vi "Last Write Block.vi"(6 "tdms file Ref":refnum<k34>, 7 "Group Name TMDS":string, 8 "error in":errorcluster, 9 "Data":waveform(dbl)[](array[waveform]), 10 "End Block?":bool, 11 "Acq and Logging Props":T1) -> (0 "error out":errorcluster, 2 "Message":string, 3 "tdms file out":refnum<k34>)   [LabVIEW 2013]
uses:
  <vilib>/Analysis/5stat.llb/RMS (DBL).vi
  <vilib>/Analysis/NI_AALPro.lvlib
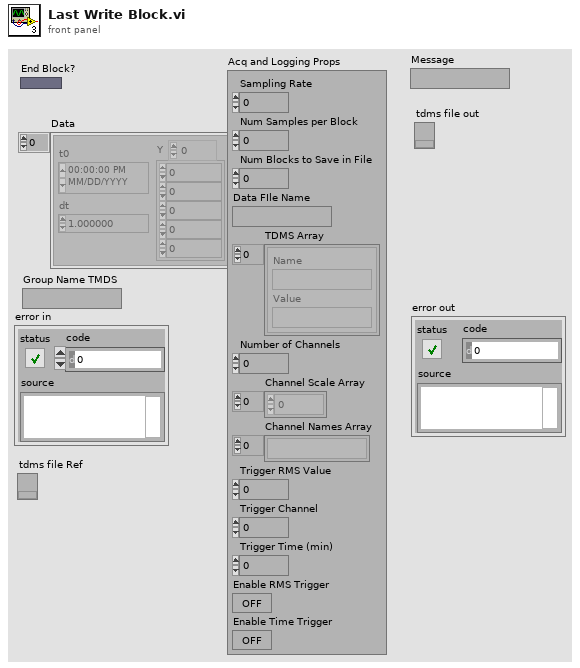
[diagram p1: front panel]
types:
  T1 = cluster{"Sampling Rate":dbl, "Num Samples per Block":i32, "Num Blocks to Save in File":i32, "Data FIle Name":string, "TDMS Array":cluster{"Name":string, "Value":string}[], "Number of Channels":i32, "Channel Scale Array":dbl[], "Channel Names Array":string[], "Trigger RMS Value":dbl, "Trigger Channel":i32, "Trigger Time (min)":i32, "Enable RMS Trigger":bool, "Enable Time Trigger":bool}
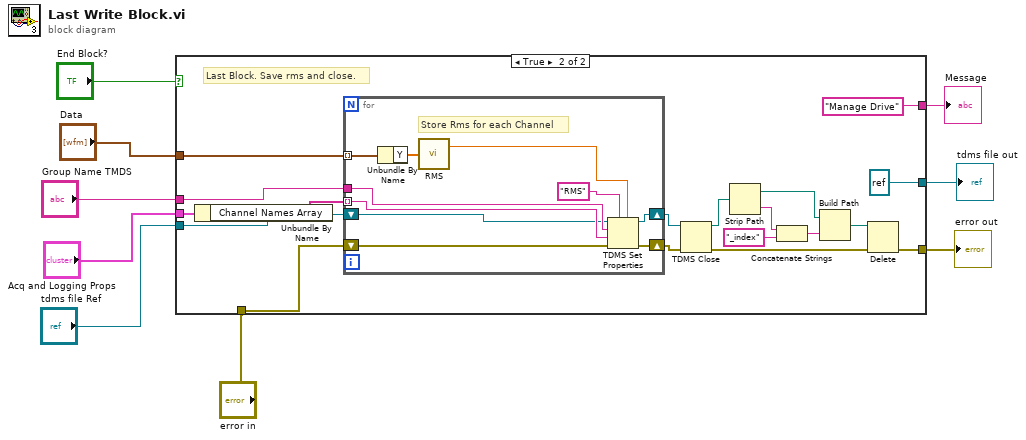
[diagram p0: block diagram]
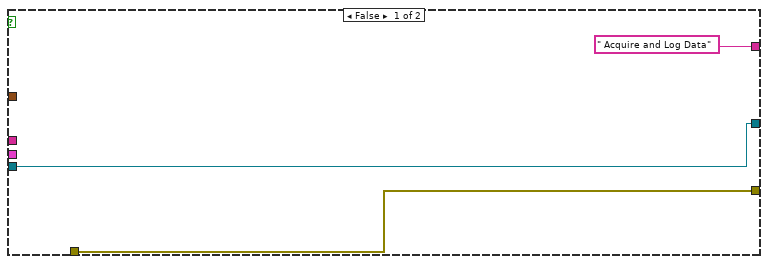
[diagram p2: hidden frame]
diagram:
  n1 = case shown="True" "End Block?" {
    tunnel: "Acq and Logging Props" -> [_ w30]
    tunnel: "Group Name TMDS" -> [_ w28]
    tunnel: "tdms file Ref" -> [w12 w27]
    tunnel: "Data" -> [_ w26]
    tunnel: [w10 w14] -> w3
    tunnel: "error in" -> [w10 w17]
    tunnel: [w12 refnum<k34> refnum ("tdms file out")] -> w2
    tunnel: [" Acquire and Log Data" ("Message") "Manage Drive" ("Message")] -> w1
    frame False {
    }
    frame True {
      # "Last Block. Save rms and close."
      n2 = Unbundle By Name(w30) -> ("Channel Names Array"=w29:string[])
      n3 = for {
        tunnel: w29 -> [w40] mode=indexing
        tunnel: w28 -> [w39]
        shift-right: [w37] -> w16
        shift-left: w27 -> [w38]
        tunnel: w26 -> [w36] mode=indexing
        shift-right: [w32] -> w19
        shift-left: w17 -> [w31]
        # "Store Rms for each Channel"
        n4 = Unbundle By Name(w36) -> ("Y"=w35:dbl[])
        n5 = call-poly <vilib>:"RMS.vi"("X"=w35) -> ("rms value"=w34:dbl)  [unwired: 1 out]
        n6 = TDMS Set Properties(5:w34, 7:"RMS" ("property names"), 8:w31, 9:w40, 10:w39, 11:w38) -> (0:w32:errorcluster, 3:w37:refnum<k34>)  [unwired: 2 out]
      }
      n7 = TDMS Close(8:w19, 11:w16) -> (0:w18:errorcluster, 3:w25:path)
      n8 = Strip Path(path=w25) -> (stripped path=w21:path, name=w24:string)
      n9 = Concatenate Strings(w24, "_index" ("string")) -> (w22:string)
      n10 = Build Path(base path=w21, name or relative path=w22) -> (appended path=w20:path)
      n11 = Delete(path (use dialog)=w20, error in=w18) -> (error out=w14:errorcluster)  [unwired: 3 in, 2 out]
    }
  }
  "error out" <- w3
  "tdms file out" <- w2
  "Message" <- w1
